vi "Simple_GPIB_MulFueV3.vi"() -> ()   [LabVIEW 2015]
panel:
  in  "Voltaje Final":i32(knob) scale=0.0..20.0
  in  "Voltaje Inicial":i32(knob) scale=0.0..20.0
  in  "Step":i32(knob) scale=0.0..5.0
  in  "Parar":bool
  out "Waveform Graph":dbl[](graph)
  out "Estado de la pantalla":string
  out "ID Fuente:":string
  out "ID Multímetro:":string
  out "ERROR":bool
  out "error out":errorcluster
  out "Array":string[](array[string])
  out "data string":string
  in  "Direcciones":i16[](array[numeric]) min=0 max=30
  # "CONTROLES"
  # "INDICADORES"
  # "MULTÍMETRO"
  # "FUENTE"
  # "V"
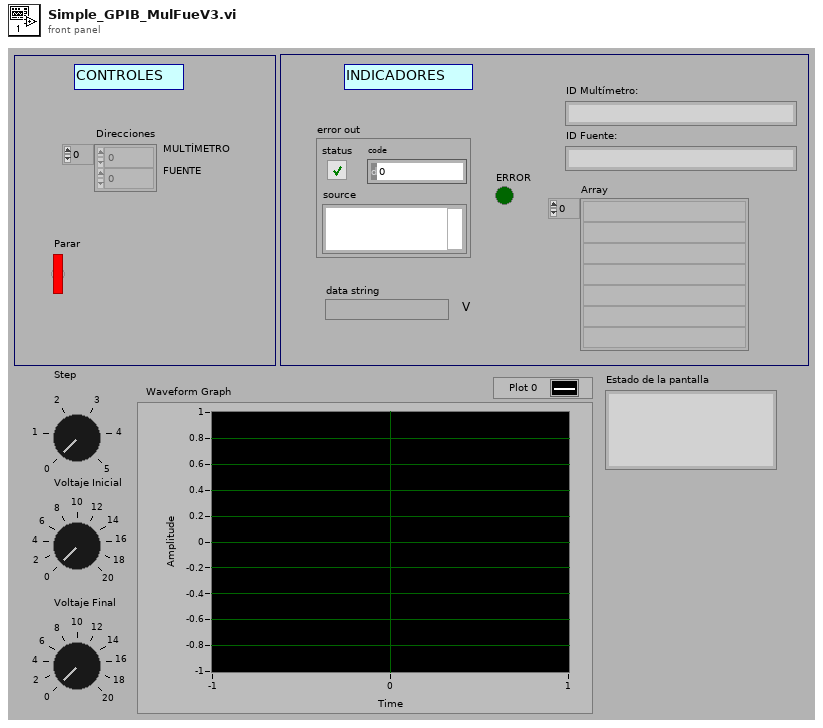
[diagram p1: front panel]
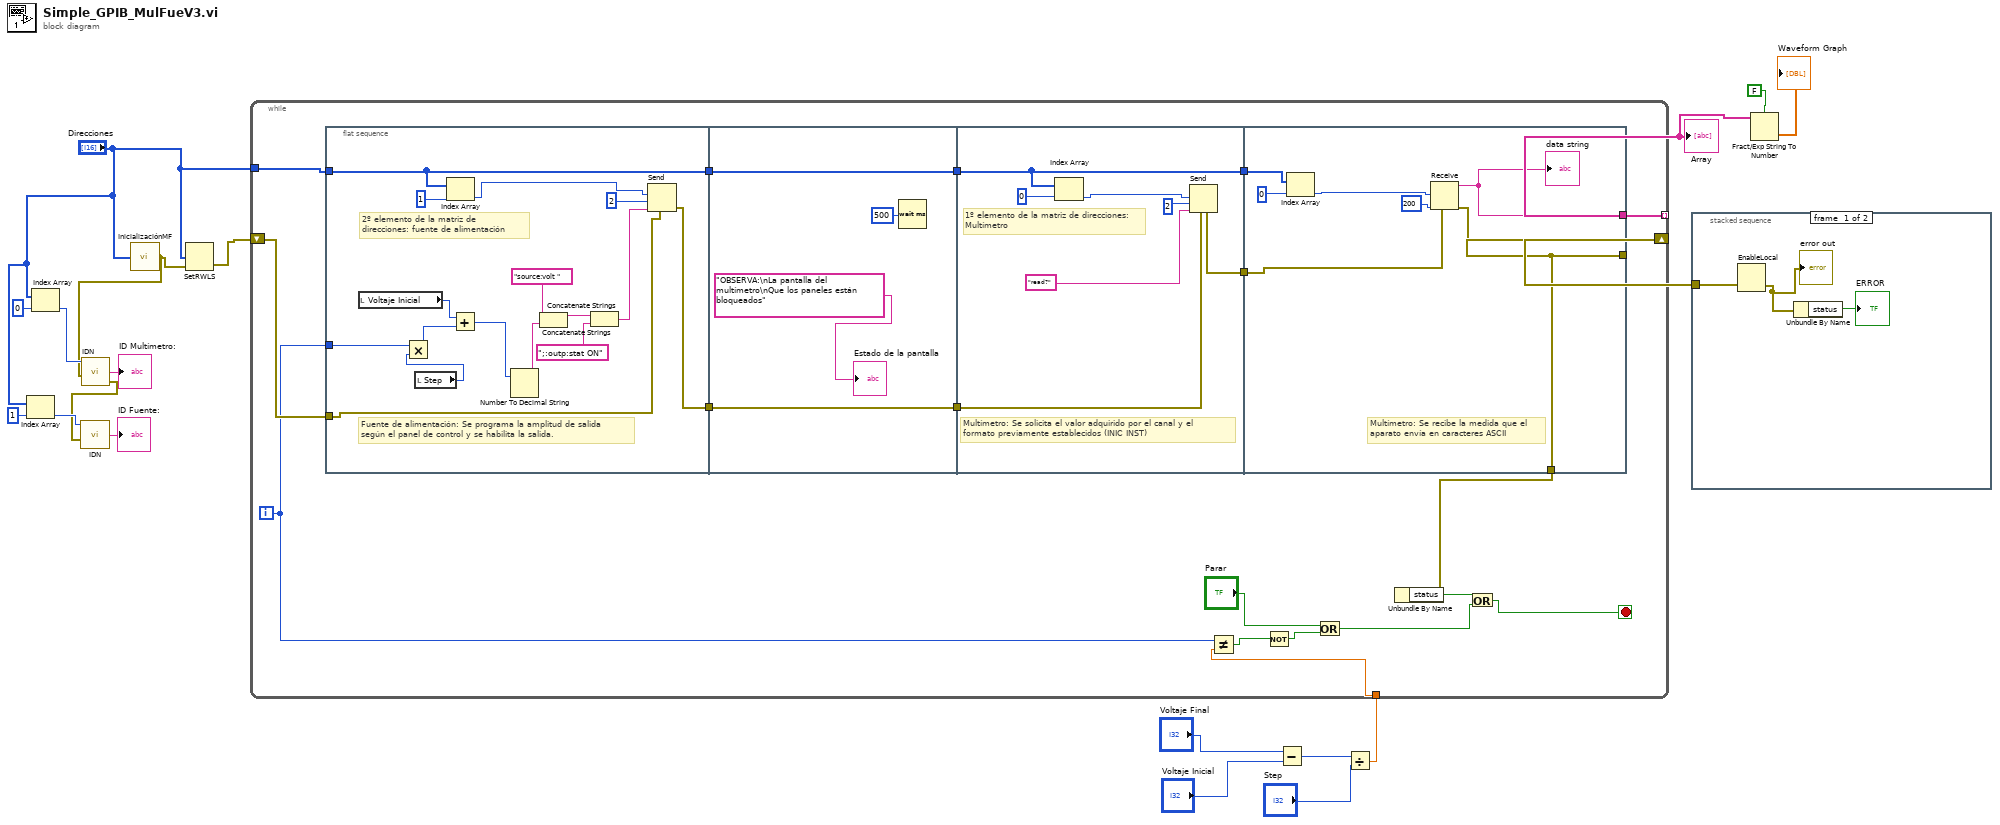
[diagram p0: block diagram]
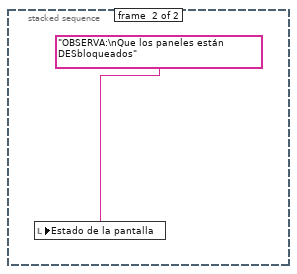
[diagram p2: hidden frame]
diagram:
  n1 = Index Array(array="Direcciones", index=1) -> (element=w11:i16)
  n2 = Index Array(array="Direcciones", index=0) -> (element=w14:i16)
  n3 = call "InicializaciónMF.vi"("Lista de Direcciones"="Direcciones") -> ("error out 2"=w10:errorcluster)
  n4 = call "IDN.vi"("error in"=w10, "Address"=w14) -> ("error out"=w9:errorcluster, "ID:"=→"ID Multímetro:":string)  [unwired: 3 in]
  n5 = call "IDN.vi"("error in"=w9, "Address"=w11) -> ("ID:"=→"ID Fuente:":string)  [unwired: 3 in, 1 out]
  n6 = SetRWLS(2:w10, 3:"Direcciones") -> (0:w18:errorcluster)  [unwired: 1 in, 1 out]
  n7 = Subtract(x="Voltaje Final", y="Voltaje Inicial") -> (x-y=w3:i32)
  n8 = Divide(x=w3, y="Step") -> (x/y=w1:dbl)
  n9 = while {
    tunnel: "Direcciones" -> [w36]
    tunnel: [w33] -> w8 mode=indexing
    shift-right: [w32] -> w19
    shift-left: w18 -> [w31]
    tunnel: w1 -> [w26]
    i -> [w28]
    stop <- w21 stop-if-true
    n10 = flat-sequence {
      tunnel: [w48] -> w38
      tunnel: w31 -> [w39]
      tunnel: w36 -> [w46]
      tunnel: [w46] -> w34
      tunnel: w28 -> [w42]
      tunnel: w38 -> [w58]
      tunnel: [w58] -> w37
      tunnel: [w57] -> w35
      tunnel: w34 -> [w57]
      tunnel: w37 -> [w59]
      tunnel: [w63] -> w30
      tunnel: w35 -> [w61]
      tunnel: [w61] -> w29
      tunnel: [w71] -> w33
      tunnel: [w67] -> w32
      tunnel: w29 -> [w68]
      tunnel: w30 -> [w66]
      tunnel: [w67] -> w23
      frame #0 {
        # "2º elemento de la matriz de direcciones: fuente de alimentación"
        # "Fuente de alimentación: Se programa la amplitud de salida según el panel de control y se habilita la salida."
        n11 = local read "Voltaje Inicial"() -> (w40:i32)
        n12 = local read "Step"() -> (w41:i32)
        n13 = Multiply(x=w42, y=w41) -> (x*y=w44:i32)
        n14 = Index Array(array=w46, index=1) -> (element=w47:i16)
        n15 = Add(x=w40, y=w44) -> (x+y=w43:i32)
        n16 = Number To Decimal String(number=w43) -> (decimal integer string=w45:string)  [unwired: 1 in]
        n17 = Concatenate Strings("source:volt ", w45) -> (w50:string)
        n18 = Concatenate Strings(w50, ";:outp:stat ON") -> (w53:string)
        n19 = Send(2:w47, 3:2, 4:w39, 5:w53) -> (8:w48:errorcluster)  [unwired: 1 in, 2 out]
      }
      frame #1 {
        n20 = Wait (ms)(milliseconds to wait=u32 500) -> ()  [unwired: 1 out]
        "Estado de la pantalla" <- "OBSERVA:\nLa pantalla del multímetro\nQue los paneles están bloqueados" ("message")
      }
      frame #2 {
        # "1º elemento de la matriz de direcciones: Multímetro"
        # "Multímetro: Se solicita el valor adquirido por el canal y el formato previamente establecidos (INIC INST)"
        n21 = Index Array(array=w61, index=0) -> (element=w60:i16)
        n22 = Send(2:w60, 3:2, 4:w59, 5:"read?") -> (8:w63:errorcluster)  [unwired: 1 in, 2 out]
      }
      frame #3 {
        # "Multímetro: Se recibe la medida que el aparato envía en caracteres ASCII"
        n23 = Index Array(array=w68, index=0) -> (element=w70:i16)
        n24 = Receive(4:w66, 6:200 ("count"), 8:w70) -> (0:w67:errorcluster, 3:w71:string)  [unwired: 2 in, 2 out]
        "data string" <- w71
      }
    }
    n25 = Not Equal?(x=w28, y=w26) -> (x != y?=w25:bool)
    n26 = Not(x=w25) -> (.not. x?=w24:bool)
    n27 = Or(x="Parar", y=w24) -> (x .or. y?=w22:bool)
    n28 = Unbundle By Name(w23) -> ("status"=w20:bool)
    n29 = Or(x=w20, y=w22) -> (x .or. y?=w21:bool)
  }
  "Array" <- w8
  n30 = stacked-sequence {
    tunnel: w19 -> [w75 _]
    frame #0 {
      n31 = EnableLocal(2:w75) -> (0:w74:errorcluster)  [unwired: 2 in, 1 out]
      "error out" <- w74
      n32 = Unbundle By Name(w74) -> ("status"=→"ERROR":bool)
    }
    frame #1 {
      n33 = local write "Estado de la pantalla"("OBSERVA:\nQue los paneles están DESbloqueados" ("message")) -> ()
    }
  }
  n34 = Fract/Exp String To Number(use system decimal point (T)=FALSE, string=w8) -> (number=→"Waveform Graph":dbl[])  [unwired: 2 in, 1 out]
